vi "mark serial.vi"(8 "error in (no error)":errorcluster, 10 "digits":u16, 11 "mode":u16) -> (0 "error out":errorcluster)   [LabVIEW 2015, in "SCANalone4x64.lvlib"]
doc: "__declspec(dllimport) void __stdcall mark_serial(unsigned short mode, unsigned short digits);"
uses:
  <userlib>/SCANalone4x64/SCANalone4x64.lvlib
  <userlib>/SCANalone4x64/SCANalone4x64.dll
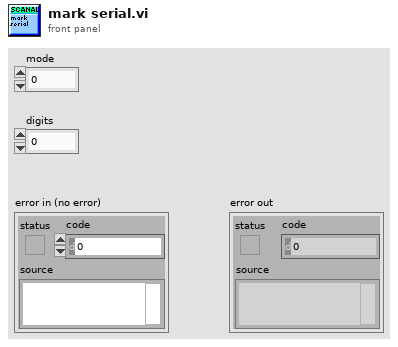
[diagram p1: front panel]
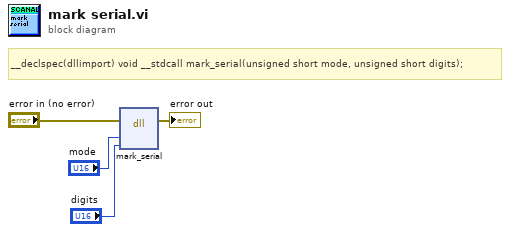
[diagram p0: block diagram]
diagram:
  # "__declspec(dllimport) void __stdcall mark_serial(unsigned short mode, unsigned short digits);"
  n1 = dll-call lib="C:/Program Files/National Instruments/LabVIEW 2015/user.lib/SCANalone4x64/SCANalone4x64.*" fn="mark_serial"(error in="error in (no error)", "mode"="mode", "digits"="digits") -> (error out=→"error out":errorcluster)  [unwired: 5 in, 1 out]
